vi "testRegStopServerOcc.vi"(8 "error in (no error)":errorcluster) -> (0 "error out":errorcluster)   [LabVIEW 2018]
doc: "Test the regStopServerOcc.vi."
uses:
  src/TcpServerBase/TcpServerBase.lvclass
  src/TcpServerBase/TcpServerBase.lvclass/TcpServerBase.ctl
  <vilib>/addons/_JKI Toolkits/Caraya/classes/Assert/Assert Equal Type_Variant.vi
  <vilib>/addons/_JKI Toolkits/Caraya/classes/Test/Test.lvclass
  <vilib>/addons/_JKI Toolkits/Caraya/classes/Assert/Assert.lvclass
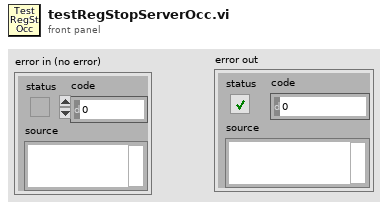
[diagram p1: front panel]
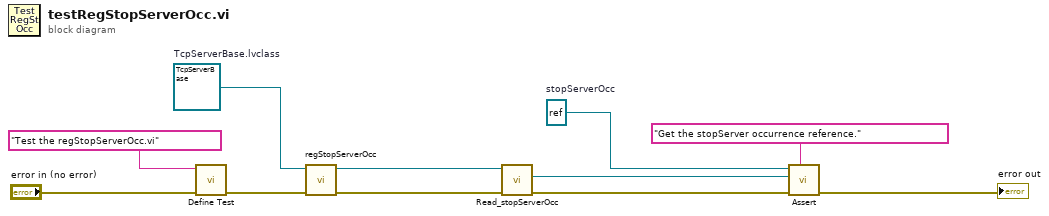
[diagram p0: block diagram]
diagram:
  w1 = refnum<k4> refnum  # stopServerOcc
  w8 = refnum<class "TcpServerBase.lvclass"> refnum  # TcpServerBase.lvclass
  n1 = call <vilib>:"Define Test.vi"("error in (no error)"="error in (no error)", "Label (VI Title)"="Test the regStopServerOcc.vi") -> ("error out"=w7:errorcluster)  [unwired: 9 in]
  n2 = call "regStopServerOcc.vi"("error in (no error)"=w7, "tcpServerBase in"=w8) -> ("error out"=w6:errorcluster, "tcpServerBase out"=w5:refnum<class "TcpServerBase.lvclass">)  [unwired: 8 in]
  n3 = call "Read_stopServerOcc.vi"("error in (no error)"=w6, "TcpServerBase in"=w5) -> ("error out"=w4:errorcluster, "stopServerOcc"=w2:refnum<k4>)  [unwired: 7 in, 1 out]
  n4 = call-poly <vilib>:"Assert.vi"("Label"="Get the stopServer occurrence reference.", "error in (no error)"=w4, "Y"=w2, "X"=w1) -> ("error out"=→"error out":errorcluster)  [unwired: 7 in]
